vi "GraphCom.vi"() -> ()   [LabVIEW 2019]
uses:
  MessageFormat1.ctl
  <vilib>/Instr/_visa.llb/VISA Configure Serial Port (Instr).vi
panel:
  out "output 3":fxp<+/-,64,32>
  out "output 2":dbl
  out "output 1":i32
  out "Slide":i32(slide) scale=0.0..100.0
  in  "Disconnect from Arduino":bool
  out "Connected":bool
  in  "Connect to Arduino":bool
  in  "VISA resource name":refnum<visa-resource-name>
  out "Rx Number":u32
  in  "stop":bool
  out "Receiving Data":bool
  out "Input buffer":string
  in  "Stop Acquisition":bool
  in  "Start Acquisition":bool
  # "Dades rebudes per UART"
  # "Dades transportades al Consumer Loop"
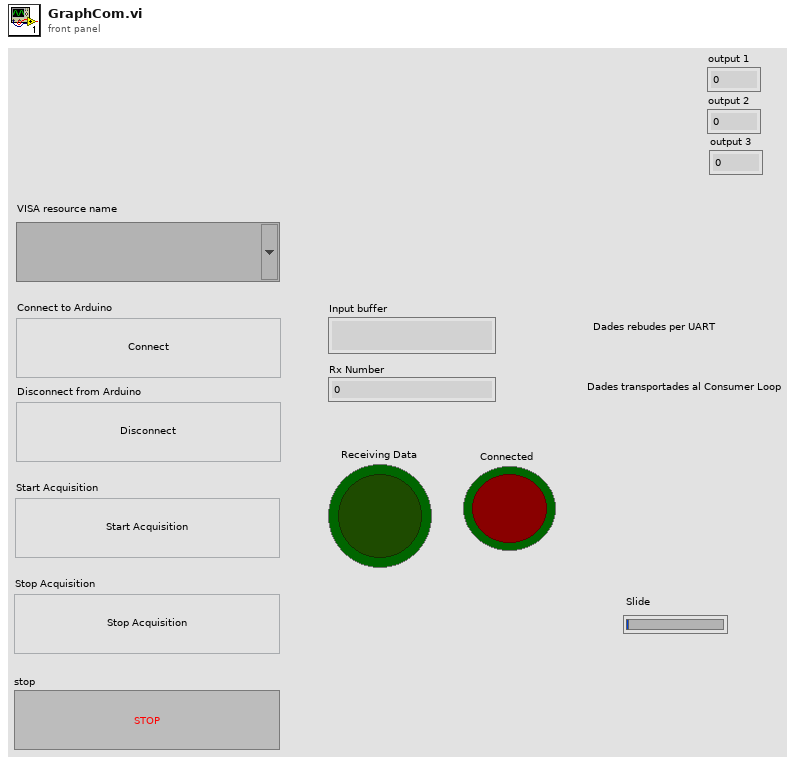
[diagram p1: front panel]
types:
  T1 = typedef "MessageFormat1.ctl" = cluster{"Consumer State":string, "RxData":string, "error constant":errorcluster, "Producer State ":string, "Numeric":dbl}
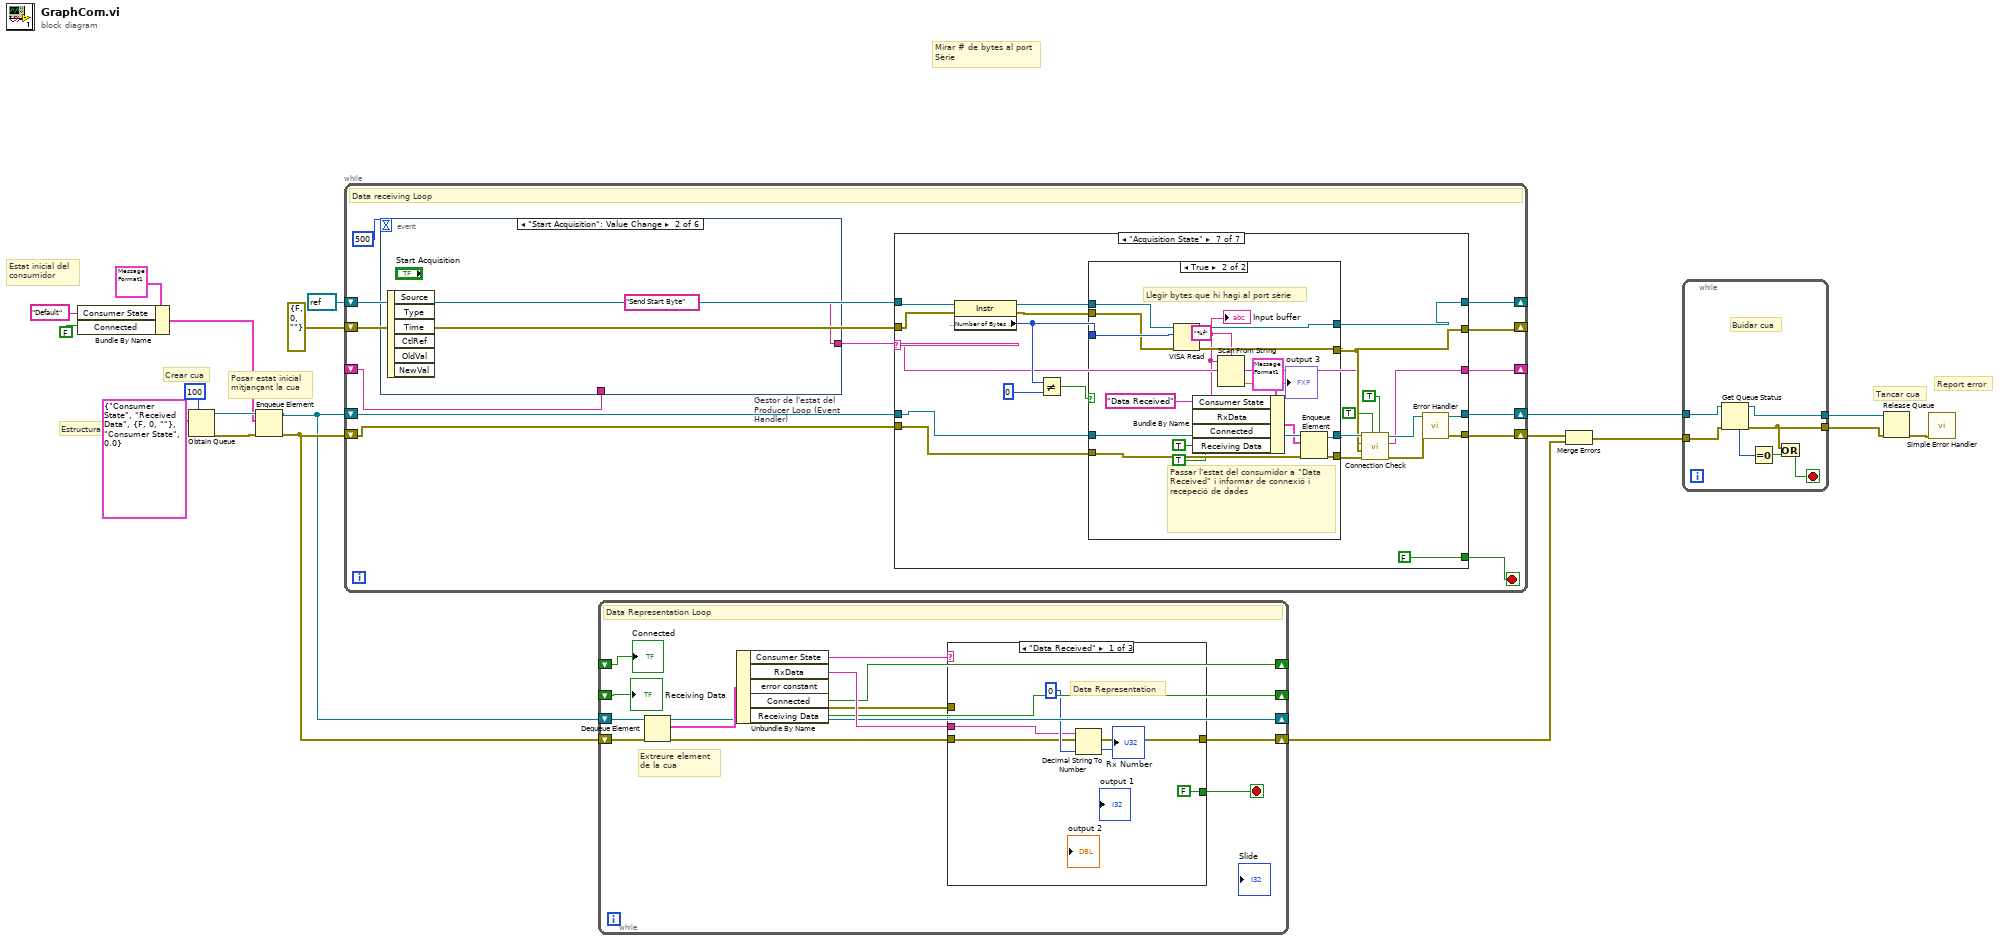
[diagram p0: block diagram]
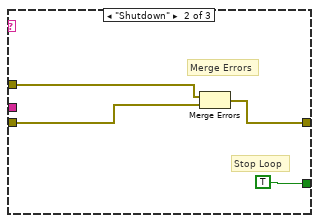
[diagram p2: hidden frame]
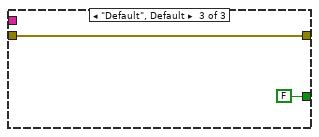
[diagram p3: hidden frame]
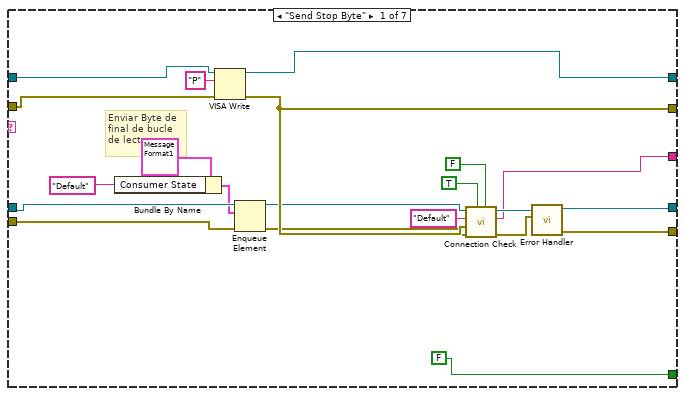
[diagram p4: hidden frame]
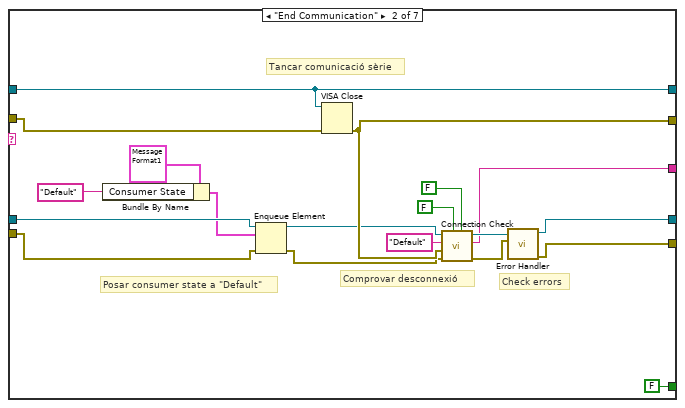
[diagram p5: hidden frame]
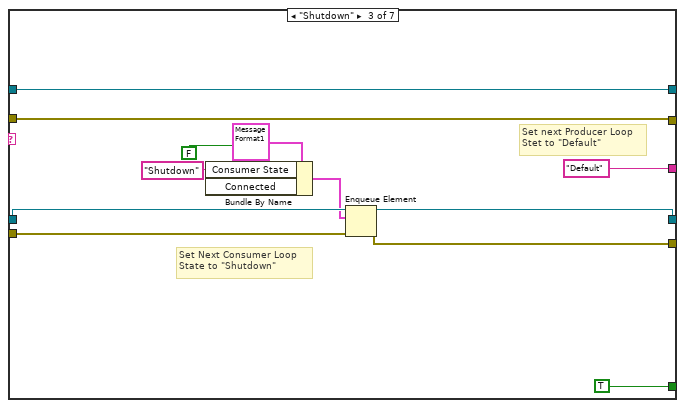
[diagram p6: hidden frame]
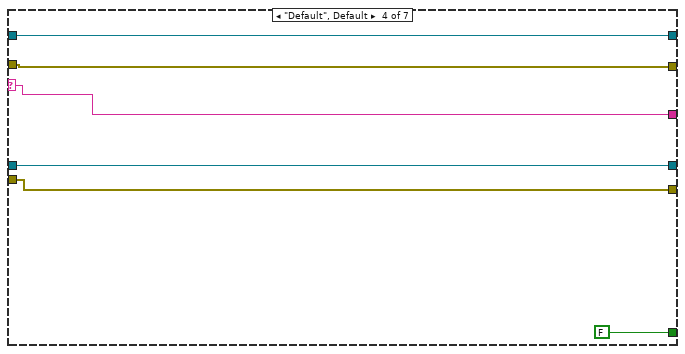
[diagram p7: hidden frame]
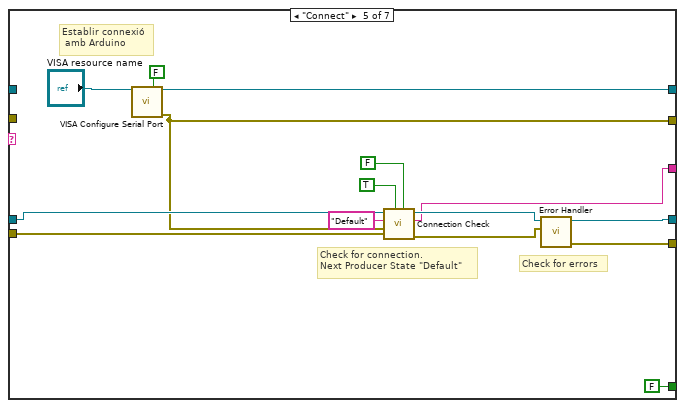
[diagram p8: hidden frame]
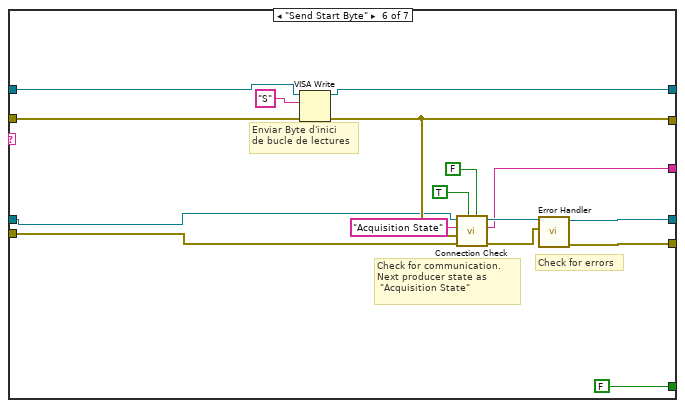
[diagram p9: hidden frame]
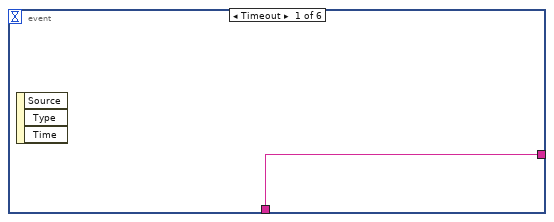
[diagram p11: hidden frame]
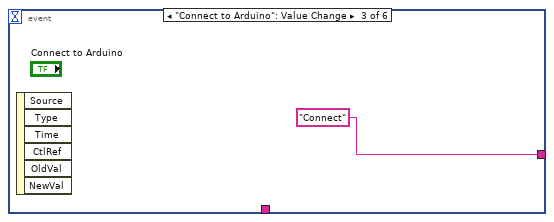
[diagram p12: hidden frame]
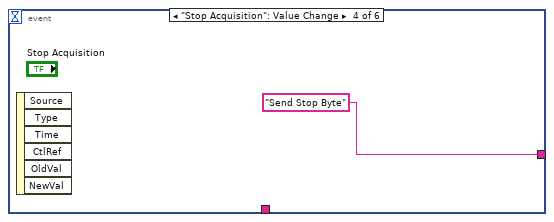
[diagram p13: hidden frame]
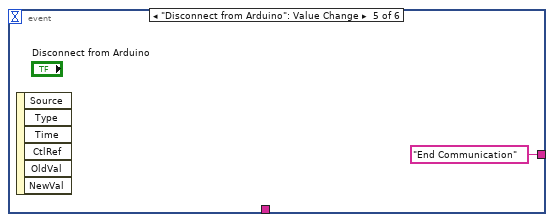
[diagram p14: hidden frame]
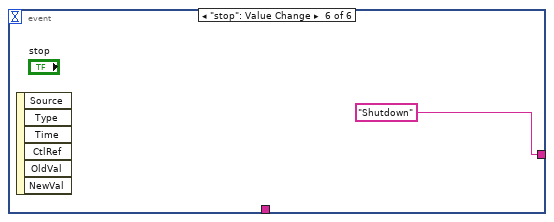
[diagram p15: hidden frame]
diagram:
  # "Tancar cua"
  # "Report error"
  # "Posar estat inicial \nmitjançant la cua"
  # "Crear cua"
  # "Mirar # de bytes al port\nSèrie"
  # "Estat inicial del \nconsumidor"
  # "Estructura de la cua"
  n1 = Bundle By Name(cluster=T1 {"Consumer State"="Consumer State", "RxData"="Received Data", "error constant"={"status"=FALSE, "code"=0, "source"=""}, "Producer State "="Consumer State", "Numeric"=0.0} ("Queue Definition"), "Consumer State"="Default", "Connected"=FALSE) -> (w10:T1)
  n2 = Obtain Queue(max queue size (-1, unlimited)=100, element data type=T1 {"Consumer State"="Consumer State", "RxData"="Received Data", "error constant"={"status"=FALSE, "code"=0, "source"=""}, "Producer State "="Consumer State", "Numeric"=0.0} ("Queue Definition")) -> (queue out=w12:refnum<queue>, error out=w15:errorcluster)  [unwired: 3 in, 1 out]
  n3 = Enqueue Element(queue=w12, element=w10, error in (no error)=w15) -> (queue out=w13:refnum<queue>, error out=w14:errorcluster)  [unwired: 1 in, 1 out]
  n4 = while {
    shift-right: [w32] -> _
    shift-left: refnum<visa-resource-name> refnum ("VISA resource name out") -> [w27]
    shift-right: [w31] -> _
    shift-left: errorcluster {"status"=FALSE, "code"=0, "source"=""} ("error out") -> [w26]
    shift-right: [w20] -> w5
    shift-left: w13 -> [w23]
    shift-right: [w21] -> w18
    shift-left: w14 -> [w24]
    shift-right: [w28] -> _
    shift-left: _ -> [w25]
    stop <- w22 stop-if-true
    # "Data receiving Loop"
    n5 = event "Gestor de l'estat del Producer Loop (Event Handler)" shown="[1] \"Start Acquisition\": Value Change" {
      selector: _ -> [_ _ _ _ _ _]
      dyn-events: _ -> [_ _ _ _ _ _]
      timeout: 500 -> [_ _ _ _ _ _]
      tunnel: [w165 "Send Start Byte" "Connect" ("f") "Send Stop Byte" "End Communication" ("Producer State Out") "Shutdown"] -> w29
      tunnel: w25 -> [w165 _ _ _ _ _]
      event Timeout {
        n6 = event-data() -> ()  [unwired: 1 in, 3 out]
      }
      event "Start Acquisition": Value Change {
        n7 = event-data() -> ()  [unwired: 1 in, 6 out]
      }
      event "Connect to Arduino": Value Change {
        n8 = event-data() -> ()  [unwired: 1 in, 6 out]
      }
      event "Stop Acquisition": Value Change {
        n9 = event-data() -> ()  [unwired: 1 in, 6 out]
      }
      event "Disconnect from Arduino": Value Change {
        n10 = event-data() -> ()  [unwired: 1 in, 6 out]
      }
      event "stop": Value Change {
        n11 = event-data() -> ()  [unwired: 1 in, 6 out]
      }
    }
    n12 = case shown="\"Acquisition State\"" w29 {
      selector: w29 -> [_ _ _ w87 _ _ w125]
      tunnel: [w49 w70 w83 w88 w102 w118 w138] -> w32
      tunnel: [w40 w63 w82 w89 w96 w112 w128] -> w31
      tunnel: [w45 w62 w77 w90 w97 w116 w127] -> w21
      tunnel: [w46 w61 w78 w85 w98 w115 w126] -> w20
      tunnel: [FALSE FALSE TRUE FALSE FALSE FALSE FALSE] -> w22
      tunnel: [w44 w64 "Default" ("f") w87 w94 w111 w124] -> w28
      tunnel: w27 -> [w50 w70 w83 w88 _ w119 w143]
      tunnel: w26 -> [w51 w71 w82 w89 _ w120 w142]
      tunnel: w24 -> [w38 w58 w76 w90 w101 w109 w136]
      tunnel: w23 -> [w37 w59 w80 w85 w100 w108 w137]
      frame "Send Stop Byte" {
        # "Enviar Byte de \nfinal de bucle \nde lectures"
        n13 = Bundle By Name(cluster=T1 {"Consumer State"="Consumer State", "RxData"="Received Data", "error constant"={"status"=FALSE, "code"=0, "source"=""}, "Producer State "="Consumer State", "Numeric"=0.0} ("Queue Definition"), "Consumer State"="Default") -> (w35:T1)
        n14 = VISA Write(VISA resource name=w50, write buffer="P", error in (no error)=w51) -> (VISA resource name out=w49:refnum<visa-resource-name>, error out=w40:errorcluster)  [unwired: 1 out]
        n15 = Enqueue Element(queue=w37, element=w35, error in (no error)=w38) -> (queue out=w36:refnum<queue>, error out=w39:errorcluster)  [unwired: 1 in, 1 out]
        n16 = call "Connection Check.vi"("Queue in"=w36, "Producer State In"="Default", "error in"=w40, "error in (no error)"=w39, "Connected"=TRUE, "Receiving Data"=FALSE) -> ("Queue out"=w48:refnum<queue>, "Producer State Out"=w44:string, "error out"=w47:errorcluster)  [unwired: 2 in]
        n17 = call "Error Handler.vi"("error in"=w47, "Queue in"=w48) -> ("error out"=w45:errorcluster, "Queue out"=w46:refnum<queue>)  [unwired: 8 in]
      }
      frame "End Communication" {
        # "Tancar comunicació sèrie"
        # "Check errors"
        # "Comprovar desconnexió"
        # "Posar consumer state a \"Default\""
        n18 = Bundle By Name(cluster=T1 {"Consumer State"="Consumer State", "RxData"="Received Data", "error constant"={"status"=FALSE, "code"=0, "source"=""}, "Producer State "="Consumer State", "Numeric"=0.0} ("Queue Definition"), "Consumer State"="Default") -> (w54:T1)
        n19 = Enqueue Element(queue=w59, element=w54, error in (no error)=w58) -> (queue out=w60:refnum<queue>, error out=w57:errorcluster)  [unwired: 1 in, 1 out]
        n20 = VISA Close(VISA resource name=w70, error in (no error)=w71) -> (error out=w63:errorcluster)
        n21 = call "Connection Check.vi"("Queue in"=w60, "Producer State In"="Default", "error in"=w63, "error in (no error)"=w57, "Connected"=FALSE, "Receiving Data"=FALSE) -> ("Queue out"=w69:refnum<queue>, "Producer State Out"=w64:string, "error out"=w68:errorcluster)  [unwired: 2 in]
        n22 = call "Error Handler.vi"("error in"=w68, "Queue in"=w69) -> ("error out"=w62:errorcluster, "Queue out"=w61:refnum<queue>)  [unwired: 8 in]
      }
      frame "Shutdown" {
        # "Set next Producer Loop\nStet to \"Default\""
        # "Set Next Consumer Loop\nState to \"Shutdown\""
        n23 = Bundle By Name(cluster=T1 {"Consumer State"="Consumer State", "RxData"="Received Data", "error constant"={"status"=FALSE, "code"=0, "source"=""}, "Producer State "="Consumer State", "Numeric"=0.0} ("Queue Definition"), "Consumer State"="Shutdown", "Connected"=FALSE) -> (w74:T1)
        n24 = Enqueue Element(queue=w80, element=w74, error in (no error)=w76) -> (queue out=w78:refnum<queue>, error out=w77:errorcluster)  [unwired: 1 in, 1 out]
      }
      frame "Default", Default {
      }
      frame "Connect" {
        # "Check for errors"
        # "Check for connection.\nNext Producer State \"Default\""
        # "Establir connexió\n amb Arduino"
        n25 = call-poly "VISA Configure Serial Port"("VISA resource name"="VISA resource name", "Enable Termination\nChar (T)"=FALSE ("Enable Termination\nChar (T)")) -> ("VISA resource name out"=w102:refnum<visa-resource-name>, "error out"=w96:errorcluster)  [unwired: 12 in]
        n26 = call "Connection Check.vi"("Queue in"=w100, "Producer State In"="Default", "error in"=w96, "error in (no error)"=w101, "Connected"=TRUE, "Receiving Data"=FALSE) -> ("Queue out"=w99:refnum<queue>, "Producer State Out"=w94:string, "error out"=w95:errorcluster)  [unwired: 2 in]
        n27 = call "Error Handler.vi"("error in"=w95, "Queue in"=w99) -> ("error out"=w97:errorcluster, "Queue out"=w98:refnum<queue>)  [unwired: 8 in]
      }
      frame "Send Start Byte" {
        # "Check for errors"
        # "Check for communication.\nNext producer state as\n \"Acquisition State\""
        # "Enviar Byte d'inici\nde bucle de lectures"
        n28 = VISA Write(VISA resource name=w119, write buffer="S", error in (no error)=w120) -> (VISA resource name out=w118:refnum<visa-resource-name>, error out=w112:errorcluster)  [unwired: 1 out]
        n29 = call "Connection Check.vi"("Queue in"=w108, "Producer State In"="Acquisition State", "error in"=w112, "error in (no error)"=w109, "Connected"=TRUE, "Receiving Data"=FALSE) -> ("Queue out"=w113:refnum<queue>, "Producer State Out"=w111:string, "error out"=w114:errorcluster)  [unwired: 2 in]
        n30 = call "Error Handler.vi"("error in"=w114, "Queue in"=w113) -> ("error out"=w116:errorcluster, "Queue out"=w115:refnum<queue>)  [unwired: 8 in]
      }
      frame "Acquisition State" {
        n31 = property class="Instr"(reference=w143, error in=w142) -> (reference out=w135:refnum<visa-resource-name>, error out=w134:errorcluster, "Serial Settings:Number of Bytes at Serial Port"=w141:u32)
        n32 = Not Equal?(x=w141, y=u32 0) -> (x != y?=w139:bool)
        n33 = case shown="True" w139 {
          tunnel: [w146 w164] -> w138
          tunnel: [w145 w155] -> w128
          tunnel: [w147 w154] -> w130
          tunnel: w141 -> [_ w162]
          tunnel: w137 -> [w147 w158]
          tunnel: w136 -> [w144 w159]
          tunnel: w135 -> [w146 w161]
          tunnel: w134 -> [w145 w160]
          tunnel: [w144 w153] -> w129
          frame False {
          }
          frame True {
            # "Passar l'estat del consumidor a \"Data Received\" i informar de connexió i recepeció de dades"
            # "Llegir bytes que hi hagi al port sèrie"
            n34 = VISA Read(VISA resource name=w161, byte count=w162, error in (no error)=w160) -> (VISA resource name out=w164:refnum<visa-resource-name>, read buffer=w148:string, error out=w155:errorcluster)  [unwired: 1 out]
            "Input buffer" <- w148
            n35 = Bundle By Name(cluster=T1 {"Consumer State"="Consumer State", "RxData"="Received Data", "error constant"={"status"=FALSE, "code"=0, "source"=""}, "Producer State "="Consumer State", "Numeric"=0.0} ("Queue Definition"), "Consumer State"="Data Received" ("Next State"), "RxData"=w148, "Connected"=TRUE, "Receiving Data"=TRUE) -> (w156:T1)
            n36 = Scan From String(format string="%f", input string=w148) -> (output 1=→"output 3":dbl)  [unwired: 3 in, 3 out]
            n37 = Enqueue Element(queue=w158, element=w156, error in (no error)=w159) -> (queue out=w154:refnum<queue>, error out=w153:errorcluster)  [unwired: 1 in, 1 out]
          }
        }
        n38 = call "Connection Check.vi"("Queue in"=w130, "Producer State In"=w125, "error in"=w128, "error in (no error)"=w129, "Connected"=TRUE, "Receiving Data"=TRUE) -> ("Queue out"=w132:refnum<queue>, "Producer State Out"=w124:string, "error out"=w131:errorcluster)  [unwired: 2 in]
        n39 = call "Error Handler.vi"("error in"=w131, "Queue in"=w132) -> ("error out"=w127:errorcluster, "Queue out"=w126:refnum<queue>)  [unwired: 8 in]
      }
    }
  }
  n40 = while {
    shift-right: [w172] -> w16
    shift-left: w14 -> [w183]
    shift-right: [w179] -> _
    shift-left: w13 -> [w184]
    shift-right: [w176] -> _
    shift-left: _ -> [w175]
    shift-right: [w174] -> _
    shift-left: _ -> [w173]
    stop <- w178 stop-if-true
    # "Extreure element \nde la cua"
    # "Data Representation Loop"
    n41 = Dequeue Element(queue=w184, error in (no error)=w183) -> (queue out=w179:refnum<queue>, element=w182:T1, error out=w171:errorcluster)  [unwired: 1 in, 1 out]
    n42 = Unbundle By Name(w182) -> ("Consumer State"=w180:string, "RxData"=w181:string, "error constant"=w177:errorcluster, "Connected"=w176:bool, "Receiving Data"=w174:bool)
    n43 = case shown="\"Data Received\"" w180 {
      tunnel: w181 -> [w185 _ _]
      tunnel: [FALSE TRUE FALSE] -> w178
      tunnel: w177 -> [_ w191 _]
      tunnel: [w186 w192 w194] -> w172
      tunnel: w171 -> [w186 w190 w194]
      frame "Data Received" {
        # "Data Representation"
        n44 = Decimal String To Number(string=w185, default (0L)=u32 0) -> (number=→"Rx Number":u32)  [unwired: 1 in, 1 out]
      }
      frame "Shutdown" {
        # "Stop Loop"
        # "Merge Errors"
        n45 = Merge Errors(w191, w190) -> (w192:errorcluster)
      }
      frame "Default", Default {
      }
    }
    "Receiving Data" <- w173
    "Connected" <- w175
  }
  n46 = Merge Errors(w18, w16) -> (w4:errorcluster)
  n47 = while {
    tunnel: w5 -> [w202]
    tunnel: w4 -> [w201]
    tunnel: [w197] -> w3
    tunnel: [w200] -> w2
    stop <- w196 stop-if-true
    # "Buidar cua"
    n48 = Get Queue Status(queue=w202, error in (no error)=w201) -> (queue out=w200:refnum<queue>, error out=w197:errorcluster, # elements in queue=w199:i32)  [unwired: 1 in, 5 out]
    n49 = Equal To 0?(x=w199) -> (x = 0?=w198:bool)
    n50 = Or(x=w197, y=w198) -> (x .or. y?=w196:bool)
  }
  n51 = Release Queue(queue=w2, error in (no error)=w3) -> (error out=w1:errorcluster)  [unwired: 1 in, 2 out]
  n52 = call <vilib>:"Simple Error Handler.vi"("error in (no error)"=w1) -> ()  [unwired: 4 in, 5 out]
